vi "HW 1 2018.vi"() -> ()   [LabVIEW 2018]
panel:
  in  "?":bool
  out "Cluster 2":T1
  in  "?":bool
  in  "?":bool
  in  "?":bool
  out "Cluster":T1
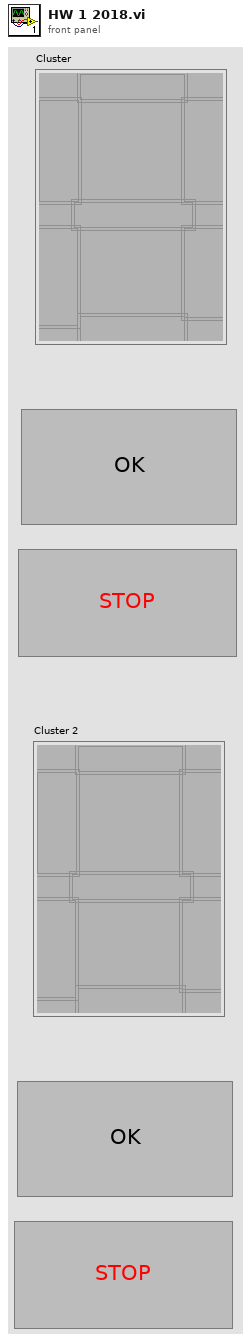
[diagram p1: front panel]
types:
  T1 = cluster{bool, bool, bool, bool, bool, bool, bool}
  T2 = cluster{"0":bool, "1":bool, "2":bool, "3":bool, " 4":bool, "5":bool, "6":bool}[]
  T3 = cluster{"0":bool, "1":bool, "2":bool, "3":bool, " 4":bool, "5":bool, "6":bool}
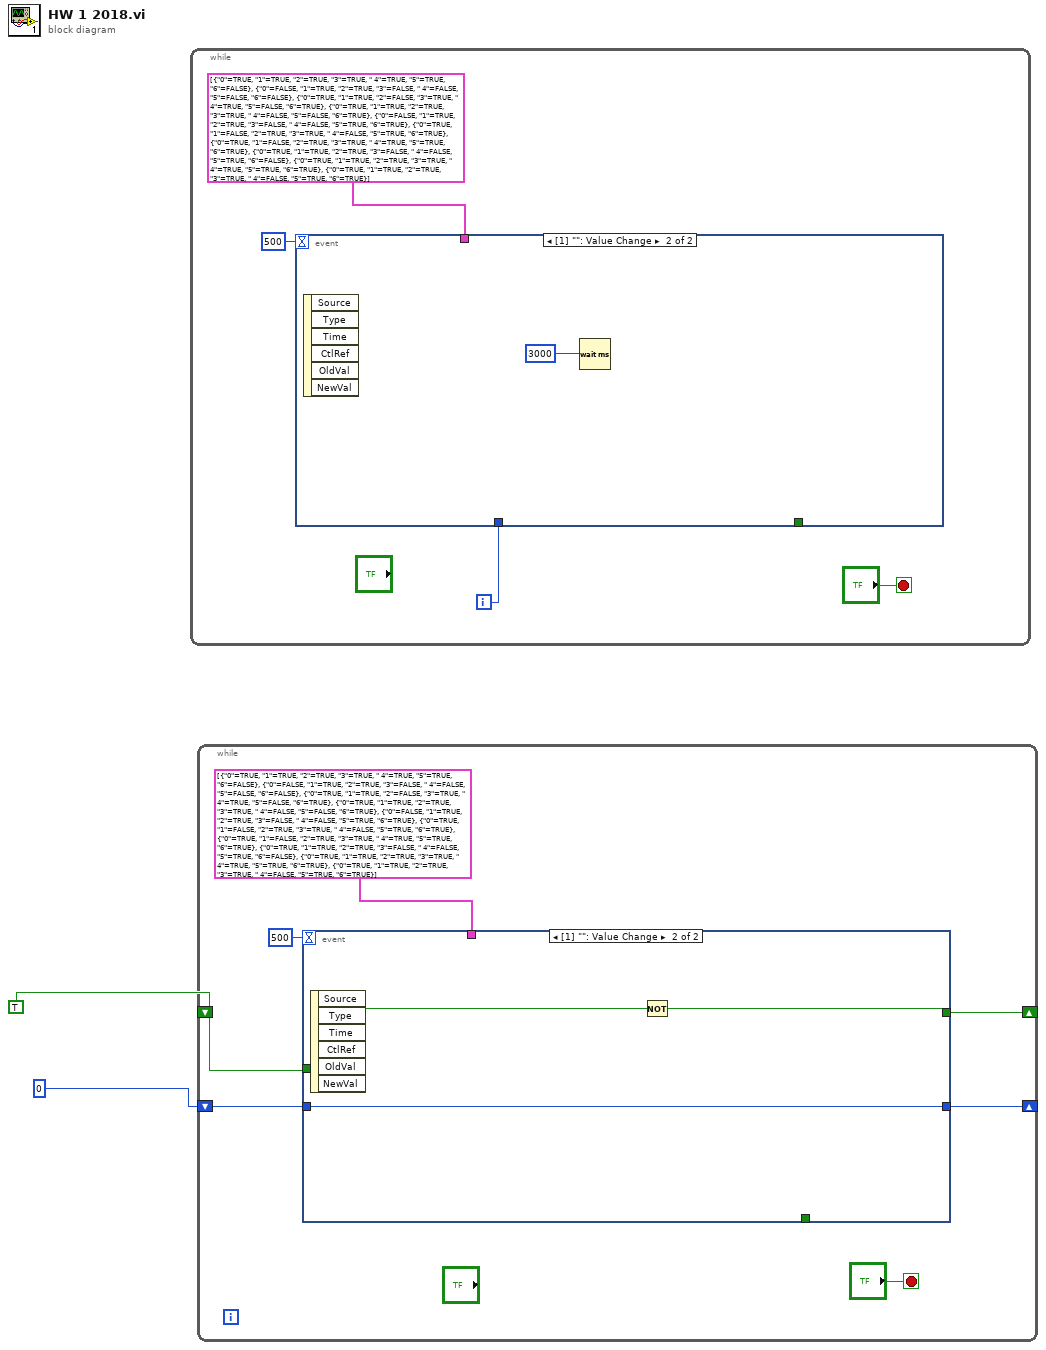
[diagram p0: block diagram]
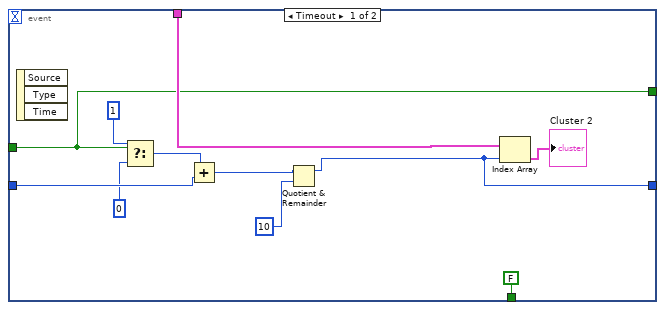
[diagram p2: hidden frame]
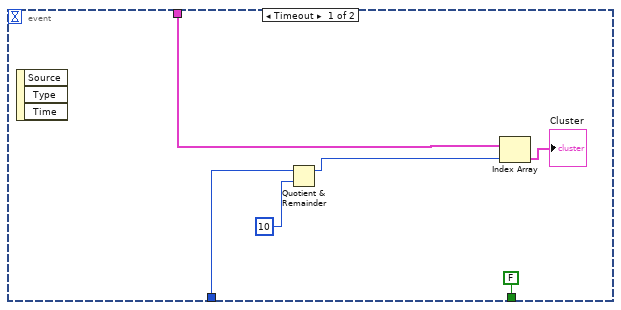
[diagram p3: hidden frame]
diagram:
  n1 = while {
    i -> [w6]
    stop <- "?" stop-if-true
    n2 = event shown="[1] \"\": Value Change" {
      selector: _ -> [_ _]
      dyn-events: _ -> [_ _]
      timeout: 500 -> [_ _]
      tunnel: w6 -> [w12 _]
      tunnel: T2 [{"0"=TRUE, "1"=TRUE, "2"=TRUE, "3"=TRUE, " 4"=TRUE, "5"=TRUE, "6"=FALSE}, {"0"=FALSE, "1"=TRUE, "2"=TRUE, "3"=FALSE, " 4"=FALSE, "5"=FALSE, "6"=FALSE}, {"0"=TRUE, "1"=TRUE, "2"=FALSE, "3"=TRUE, " 4"=TRUE, "5"=FALSE, "6"=TRUE}, {"0"=TRUE, "1"=TRUE, "2"=TRUE, "3"=TRUE, " 4"=FALSE, "5"=FALSE, "6"=TRUE}, {"0"=FALSE, "1"=TRUE, "2"=TRUE, "3"=FALSE, " 4"=FALSE, "5"=TRUE, "6"=TRUE}, {"0"=TRUE, "1"=FALSE, "2"=TRUE, "3"=TRUE, " 4"=FALSE, "5"=TRUE, "6"=TRUE}, {"0"=TRUE, "1"=FALSE, "2"=TRUE, "3"=TRUE, " 4"=TRUE, "5"=TRUE, "6"=TRUE}, {"0"=TRUE, "1"=TRUE, "2"=TRUE, "3"=FALSE, " 4"=FALSE, "5"=TRUE, "6"=FALSE}, {"0"=TRUE, "1"=TRUE, "2"=TRUE, "3"=TRUE, " 4"=TRUE, "5"=TRUE, "6"=TRUE}, {"0"=TRUE, "1"=TRUE, "2"=TRUE, "3"=TRUE, " 4"=FALSE, "5"=TRUE, "6"=TRUE}] -> [w11 _]
      tunnel: [FALSE ("OK Button") _] -> _
      event Timeout {
        n3 = event-data() -> ()  [unwired: 1 in, 3 out]
        n4 = Quotient & Remainder(x=w12, y=10) -> (x-y*floor(x/y)=w8:i32)  [unwired: 1 out]
        n5 = Index Array(array=w11, index=w8) -> (element=→"Cluster":T3)
      }
      event Value Change {
        n6 = event-data() -> ()  [unwired: 1 in, 6 out]
        n7 = Wait (ms)(milliseconds to wait=u32 3000 ("millisecond timer value")) -> ()  [unwired: 1 out]
      }
    }
  }
  n8 = while {
    shift-right: [w16] -> _
    shift-left: 0 -> [w17]
    shift-right: [w14] -> _
    shift-left: TRUE -> [w15]
    stop <- "?" stop-if-true
    n9 = event shown="[1] \"\": Value Change" {
      selector: _ -> [_ _]
      dyn-events: _ -> [_ _]
      timeout: 500 -> [_ _]
      tunnel: T2 [{"0"=TRUE, "1"=TRUE, "2"=TRUE, "3"=TRUE, " 4"=TRUE, "5"=TRUE, "6"=FALSE}, {"0"=FALSE, "1"=TRUE, "2"=TRUE, "3"=FALSE, " 4"=FALSE, "5"=FALSE, "6"=FALSE}, {"0"=TRUE, "1"=TRUE, "2"=FALSE, "3"=TRUE, " 4"=TRUE, "5"=FALSE, "6"=TRUE}, {"0"=TRUE, "1"=TRUE, "2"=TRUE, "3"=TRUE, " 4"=FALSE, "5"=FALSE, "6"=TRUE}, {"0"=FALSE, "1"=TRUE, "2"=TRUE, "3"=FALSE, " 4"=FALSE, "5"=TRUE, "6"=TRUE}, {"0"=TRUE, "1"=FALSE, "2"=TRUE, "3"=TRUE, " 4"=FALSE, "5"=TRUE, "6"=TRUE}, {"0"=TRUE, "1"=FALSE, "2"=TRUE, "3"=TRUE, " 4"=TRUE, "5"=TRUE, "6"=TRUE}, {"0"=TRUE, "1"=TRUE, "2"=TRUE, "3"=FALSE, " 4"=FALSE, "5"=TRUE, "6"=FALSE}, {"0"=TRUE, "1"=TRUE, "2"=TRUE, "3"=TRUE, " 4"=TRUE, "5"=TRUE, "6"=TRUE}, {"0"=TRUE, "1"=TRUE, "2"=TRUE, "3"=TRUE, " 4"=FALSE, "5"=TRUE, "6"=TRUE}] -> [w31 _]
      tunnel: [FALSE ("OK Button") _] -> _
      tunnel: w17 -> [w26 w34]
      tunnel: [w24 w34] -> w16
      tunnel: w15 -> [w21 w32]
      tunnel: [w21 w33] -> w14
      event Timeout {
        n10 = event-data() -> ()  [unwired: 1 in, 3 out]
        n11 = Select(t=1, s=w21, f=0) -> (s? t:f=w27:i32)
        n12 = Add(x=w27, y=w26) -> (x+y=w25:i32)
        n13 = Quotient & Remainder(x=w25, y=10) -> (x-y*floor(x/y)=w24:i32)  [unwired: 1 out]
        n14 = Index Array(array=w31, index=w24) -> (element=→"Cluster 2":T3)
      }
      event Value Change {
        n15 = event-data() -> ()  [unwired: 1 in, 6 out]
        n16 = Not(x=w32) -> (.not. x?=w33:bool)
      }
    }
  }
